vi "image_type_number_conversion.vi"(10 "input number":u16) -> (3 "converted number":u16)   [LabVIEW 2011]
doc: "Converts a number/array of a certain type to U8, U16 or I16 values in agreement with the image type that is set in the global variable"
uses:
  global_vars.vi
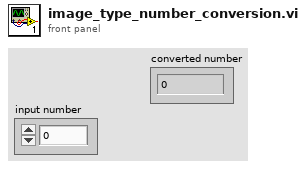
[diagram p1: front panel]
types:
  T1 = typedef "Image Type" = u32
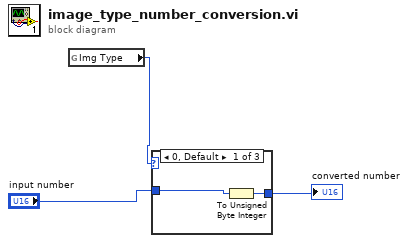
[diagram p0: block diagram]
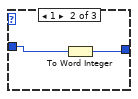
[diagram p2: hidden frame]
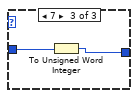
[diagram p3: hidden frame]
diagram:
  n1 = global read "global_vars.vi" "Img Type"() -> (w1:T1)
  n2 = case shown="0, Default" w1 {
    tunnel: "input number" -> [w5 w7 w9]
    tunnel: [w4 w6 w8] -> w3
    frame 0, Default {
      n3 = To Unsigned Byte Integer(number=w5) -> (unsigned 8bit integer=w4:u8)
    }
    frame 1 {
      n4 = To Word Integer(number=w7) -> (16bit integer=w6:i16)
    }
    frame 7 {
      n5 = To Unsigned Word Integer(number=w9) -> (unsigned 16bit integer=w8:u16)
    }
  }
  "converted number" <- w3
